vi "Generate Topic Rule Action JSON.vi"(11 "Topic Rule":T1) -> (3 "Action JSON":string)   [LabVIEW 2015, in "NI_AWS_IoT.lvlib"]
uses:
  NI_AWS_IoT.lvlib
  Topic Rule.ctl
  CloudWatch Alarm.ctl
  CloudWatch Metric.ctl
  DynamoDB.ctl
  DynamoDBv2.ctl
  Elasticsearch.ctl
  Firehose.ctl
  Kinesis.ctl
  Lambda.ctl
  Republish.ctl
  S3.ctl
  SNS.ctl
  SQS.ctl
  JSON Parsing/NI_JSON Parsing.lvlib
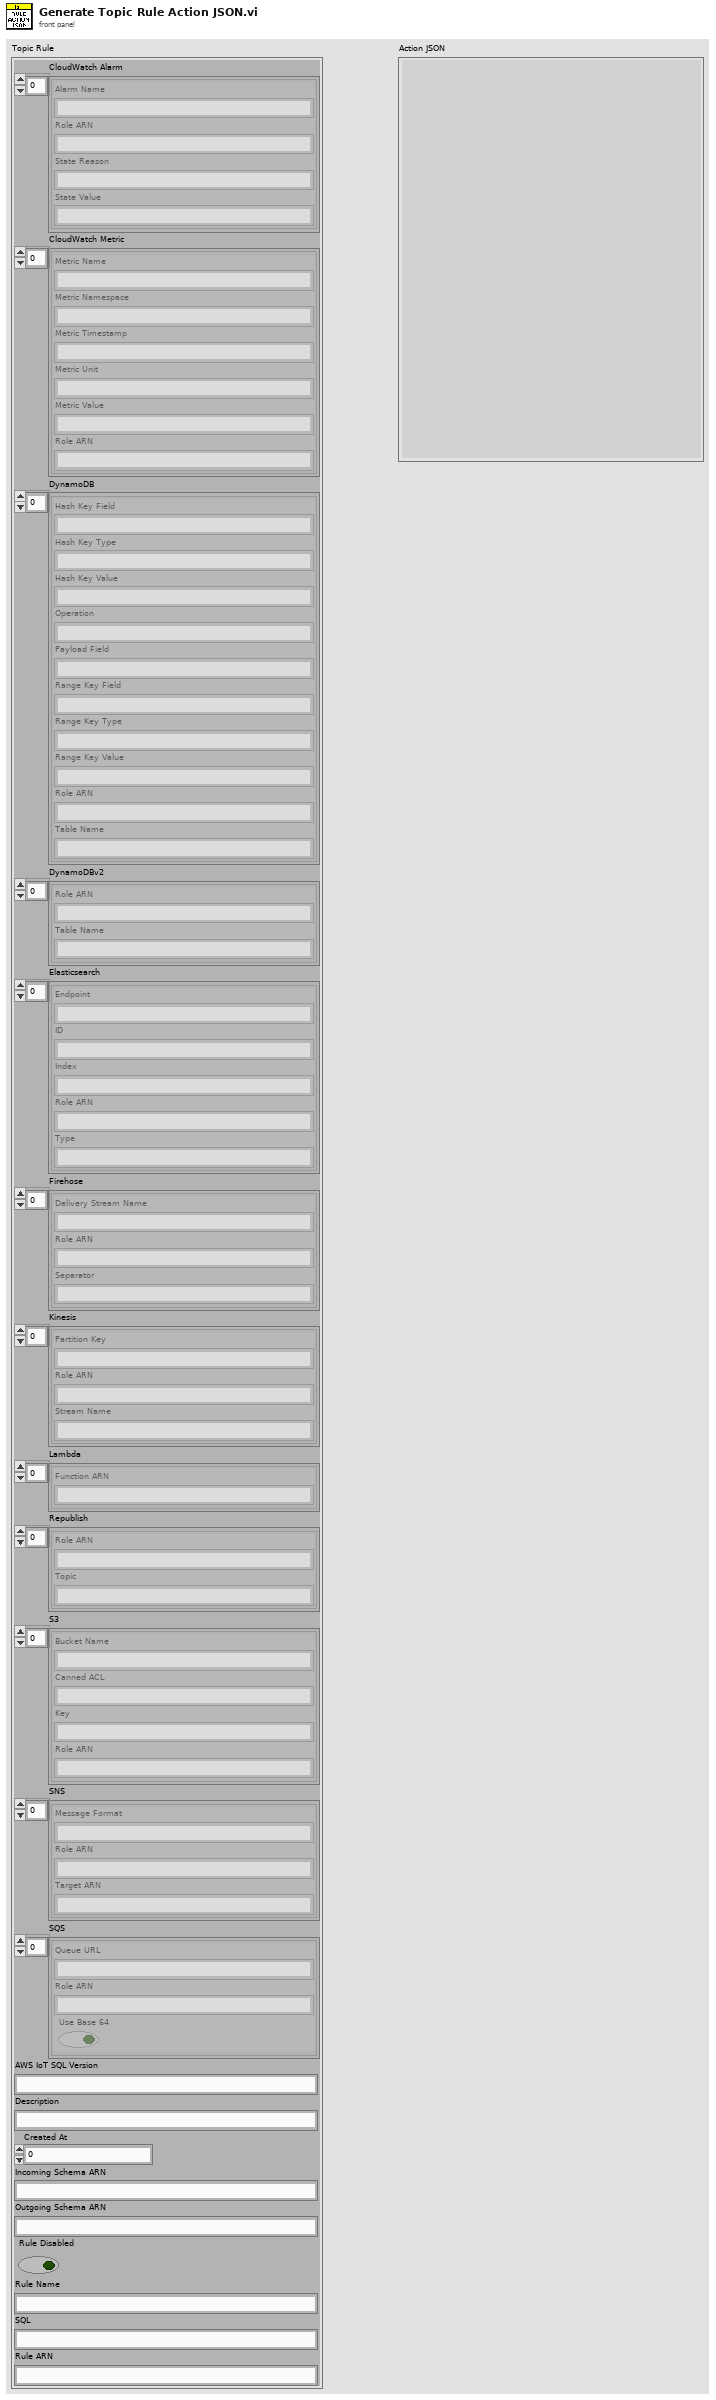
[diagram p1: front panel]
types:
  T1 = typedef "NI_AWS_IoT.lvlib/Topic Rule.ctl" = cluster{"CloudWatch Alarm":T2[], "CloudWatch Metric":T3[], "DynamoDB":T4[], "DynamoDBv2":T5[], "Elasticsearch":T6[], "Firehose":T7[], "Kinesis":T8[], "Lambda":T9[], "Republish":T10[], "S3":T11[], "SNS":T12[], "SQS":T13[], "AWS IoT SQL Version":string, "Description":string, "Created At":u64, "Incoming Schema ARN":string, "Outgoing Schema ARN":string, "Rule Disabled":bool, "Rule Name":string, "SQL":string, "Rule ARN":string}
  T2 = typedef "NI_AWS_IoT.lvlib/CloudWatch Alarm.ctl" = cluster{"Alarm Name":string, "Role ARN":string, "State Reason":string, "State Value":string}
  T3 = typedef "NI_AWS_IoT.lvlib/CloudWatch Metric.ctl" = cluster{"Metric Name":string, "Metric Namespace":string, "Metric Timestamp":string, "Metric Unit":string, "Metric Value":string, "Role ARN":string}
  T4 = typedef "NI_AWS_IoT.lvlib/DynamoDB.ctl" = cluster{"Hash Key Field":string, "Hash Key Type":string, "Hash Key Value":string, "Operation":string, "Payload Field":string, "Range Key Field":string, "Range Key Type":string, "Range Key Value":string, "Role ARN":string, "Table Name":string}
  T5 = typedef "NI_AWS_IoT.lvlib/DynamoDBv2.ctl" = cluster{"Role ARN":string, "Table Name":string}
  T6 = typedef "NI_AWS_IoT.lvlib/Elasticsearch.ctl" = cluster{"Endpoint":string, "ID":string, "Index":string, "Role ARN":string, "Type":string}
  T7 = typedef "NI_AWS_IoT.lvlib/Firehose.ctl" = cluster{"Delivery Stream Name":string, "Role ARN":string, "Separator":string}
  T8 = typedef "NI_AWS_IoT.lvlib/Kinesis.ctl" = cluster{"Partition Key":string, "Role ARN":string, "Stream Name":string}
  T9 = typedef "NI_AWS_IoT.lvlib/Lambda.ctl" = cluster{"Function ARN":string}
  T10 = typedef "NI_AWS_IoT.lvlib/Republish.ctl" = cluster{"Role ARN":string, "Topic":string}
  T11 = typedef "NI_AWS_IoT.lvlib/S3.ctl" = cluster{"Bucket Name":string, "Canned ACL":string, "Key":string, "Role ARN":string}
  T12 = typedef "NI_AWS_IoT.lvlib/SNS.ctl" = cluster{"Message Format":string, "Role ARN":string, "Target ARN":string}
  T13 = typedef "NI_AWS_IoT.lvlib/SQS.ctl" = cluster{"Queue URL":string, "Role ARN":string, "Use Base 64":bool}
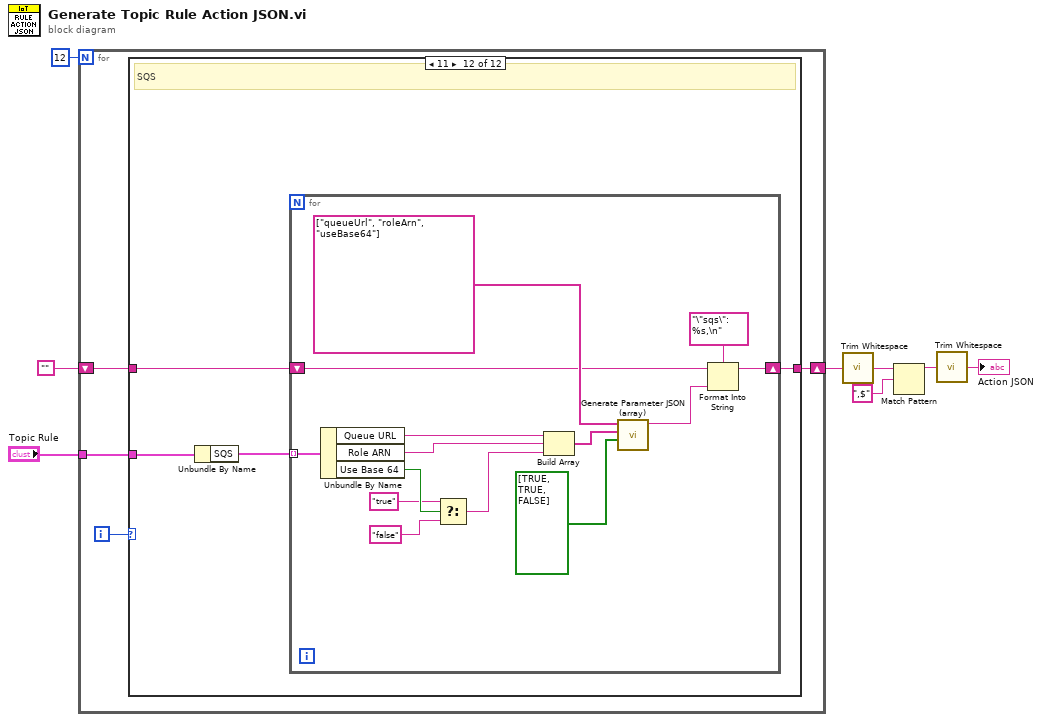
[diagram p0: block diagram]
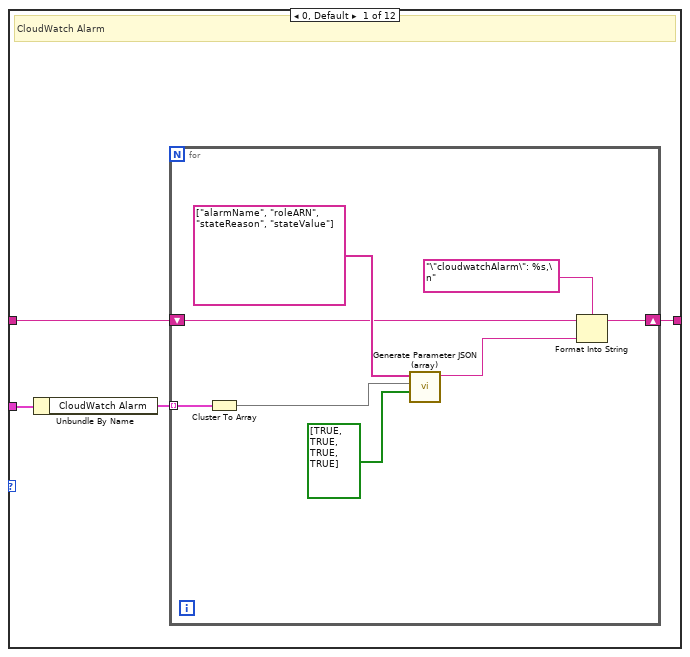
[diagram p2: hidden frame]
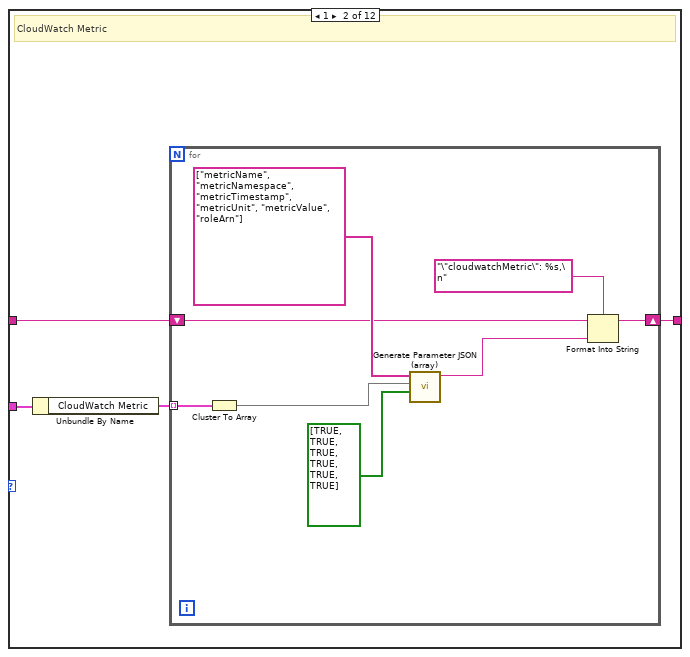
[diagram p3: hidden frame]
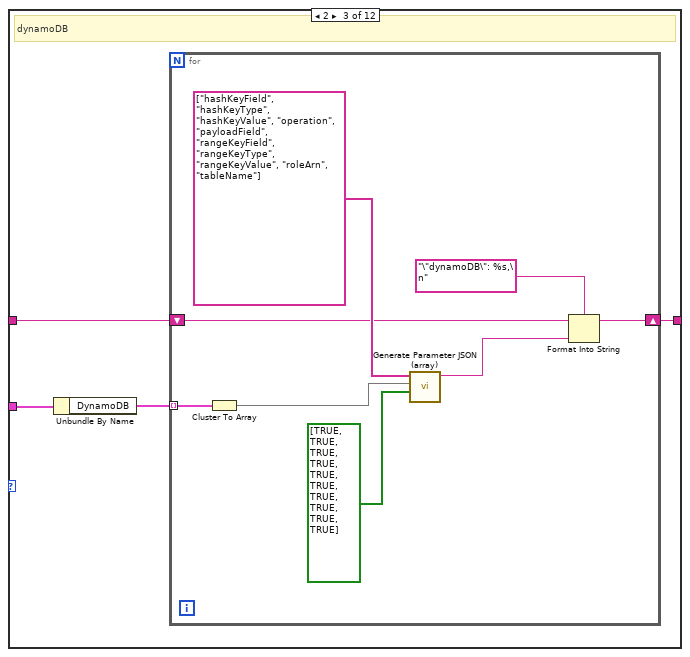
[diagram p4: hidden frame]
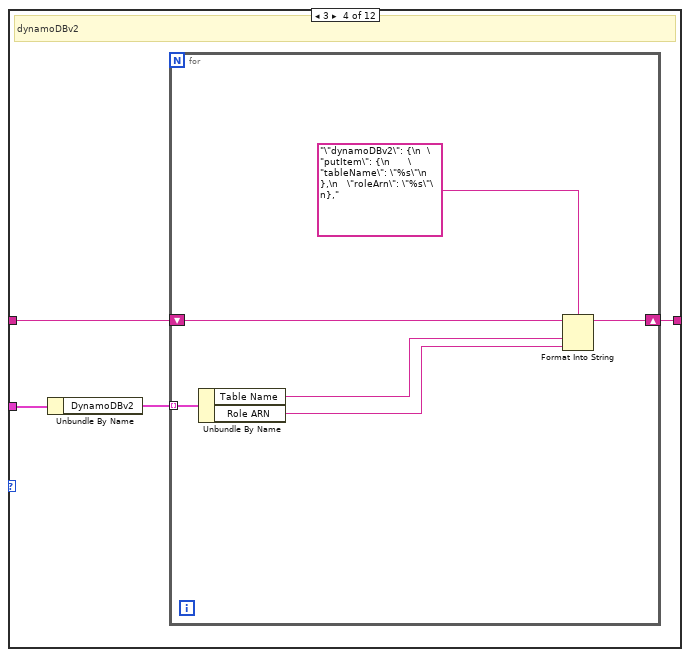
[diagram p5: hidden frame]
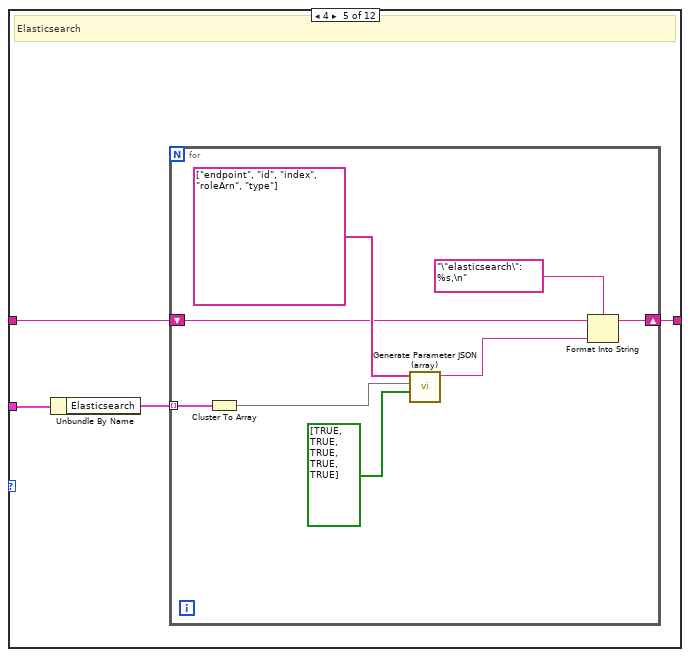
[diagram p6: hidden frame]
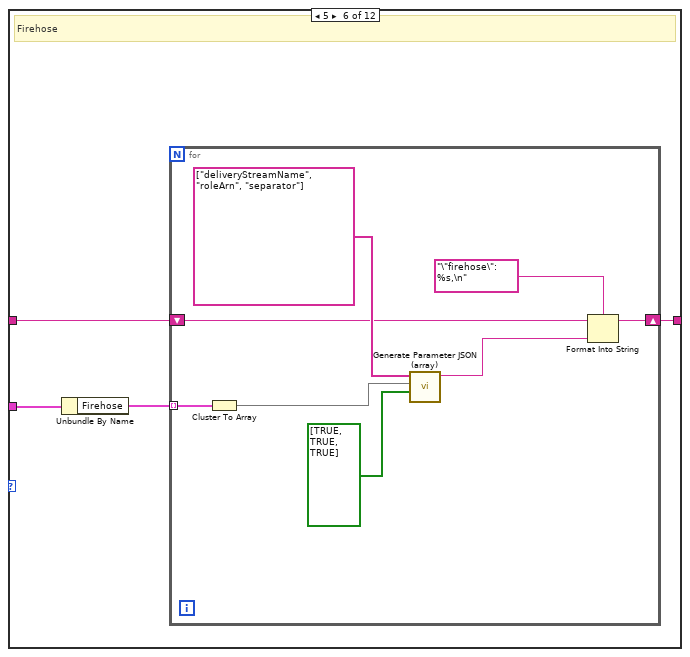
[diagram p7: hidden frame]
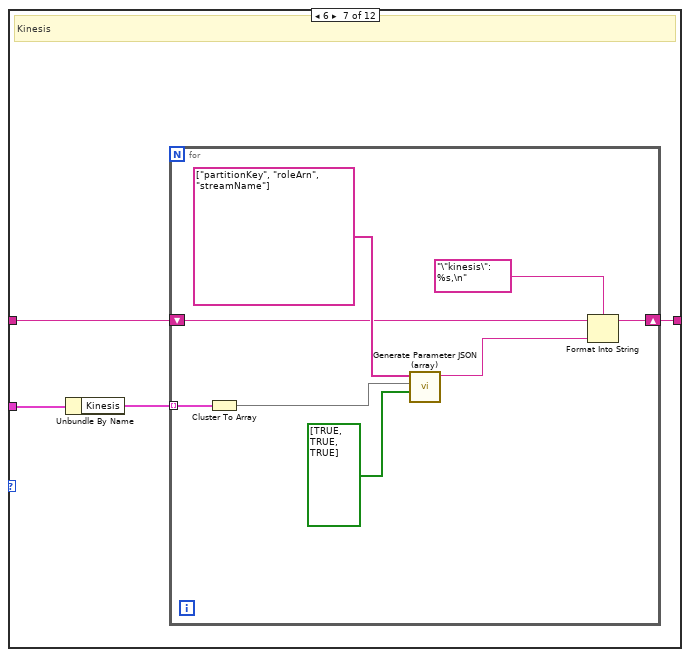
[diagram p8: hidden frame]
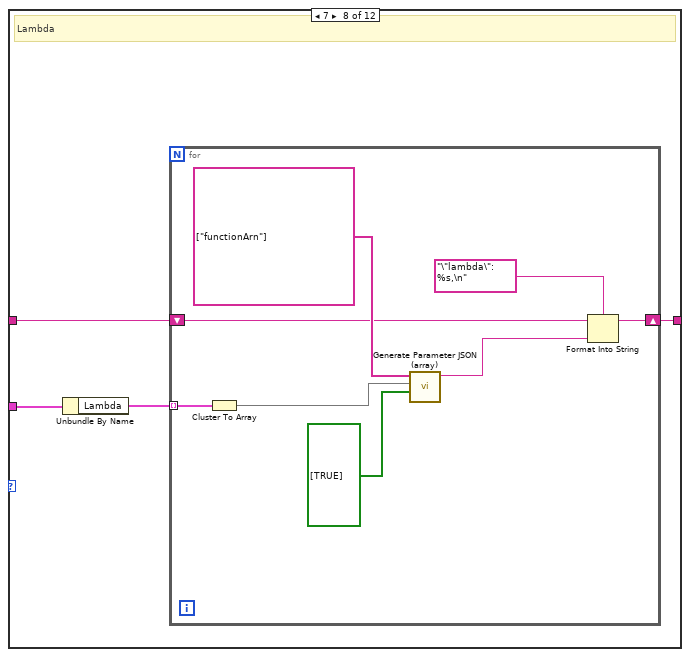
[diagram p9: hidden frame]
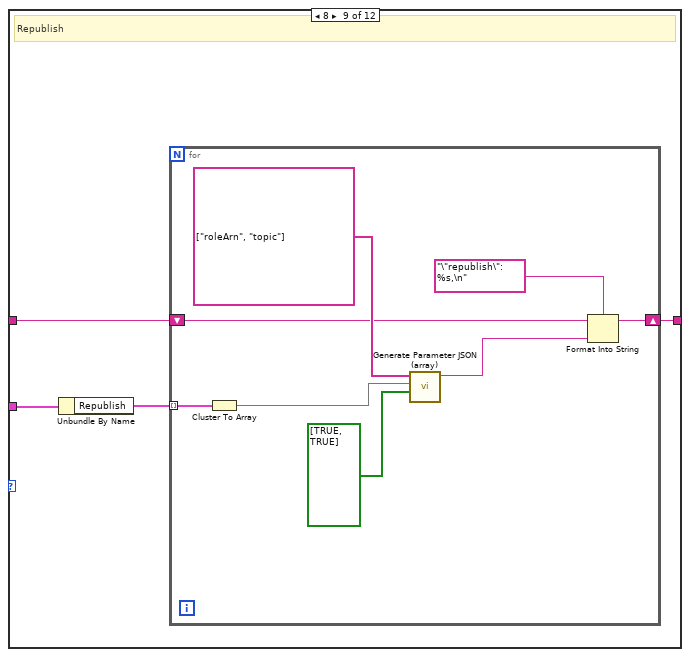
[diagram p10: hidden frame]
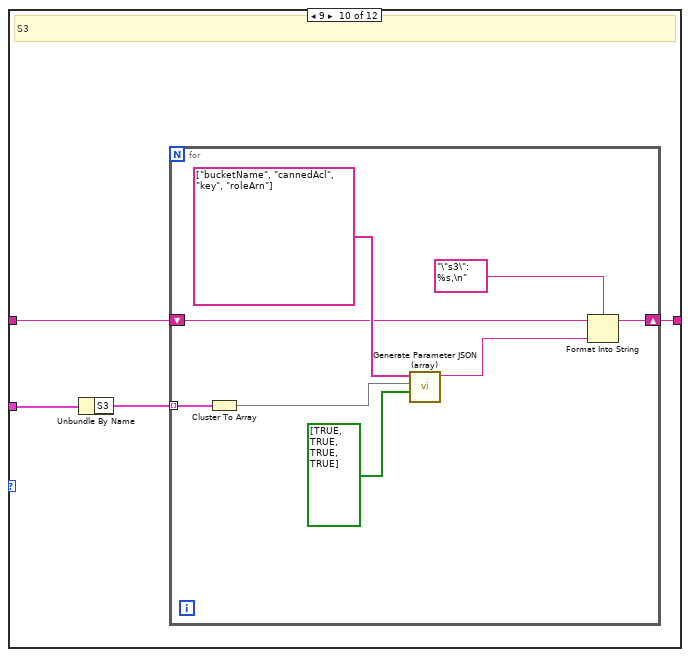
[diagram p11: hidden frame]
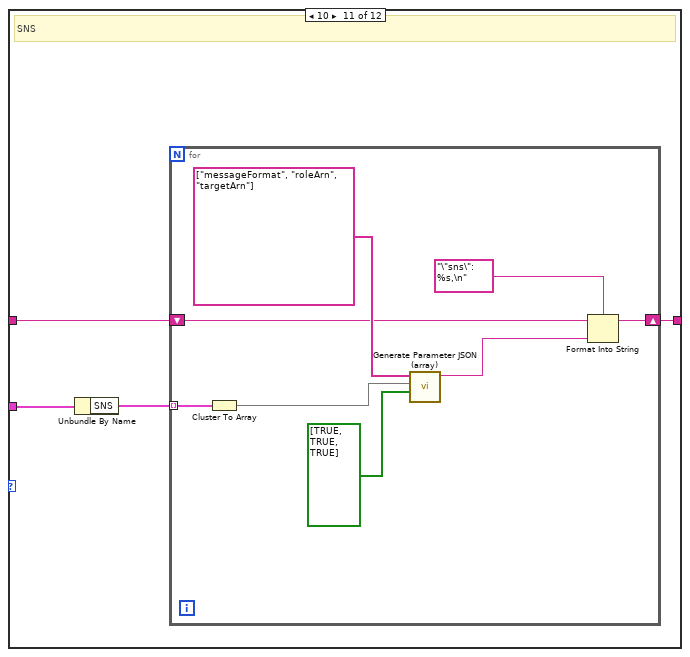
[diagram p12: hidden frame]
diagram:
  n1 = for {
    N: 12 -> [_]
    shift-right: [w9] -> w6
    shift-left: "" -> [w11]
    tunnel: "Topic Rule" -> [w10]
    i -> [w12]
    n2 = case shown="11" w12 {
      tunnel: w11 -> [w14 w26 w38 w50 w60 w72 w84 w96 w108 w120 w132 w144]
      tunnel: w10 -> [w16 w28 w40 w52 w62 w74 w86 w98 w110 w122 w134 w146]
      tunnel: [w13 w25 w37 w49 w59 w71 w83 w95 w107 w119 w131 w143] -> w9
      frame 0, Default {
        # "CloudWatch Alarm"
        n3 = Unbundle By Name(w16) -> ("CloudWatch Alarm"=w15:T2[])
        n4 = for {
          tunnel: w15 -> [w24] mode=indexing
          shift-right: [w19] -> w13
          shift-left: w14 -> [w20]
          n5 = Cluster To Array(cluster=w24) -> (array=w22:string[])
          n6 = call "Generate Parameter JSON (array).vi"("Value in Quotes"=bool[] [TRUE, TRUE, TRUE, TRUE], "Parameter Values"=w22, "Parameter Names"=string[] ["alarmName", "roleARN", "stateReason", "stateValue"]) -> ("Parameter Array JSON"=w17:string)  [unwired: 8 in]
          n7 = Format Into String(format string="\"cloudwatchAlarm\": %s,\n", initial string=w20, w17) -> (resulting string=w19:string)  [unwired: 1 in, 1 out]
        }
      }
      frame 1 {
        # "CloudWatch Metric"
        n8 = Unbundle By Name(w28) -> ("CloudWatch Metric"=w27:T3[])
        n9 = for {
          tunnel: w27 -> [w36] mode=indexing
          shift-right: [w30] -> w25
          shift-left: w26 -> [w32]
          n10 = Cluster To Array(cluster=w36) -> (array=w34:string[])
          n11 = call "Generate Parameter JSON (array).vi"("Value in Quotes"=bool[] [TRUE, TRUE, TRUE, TRUE, TRUE, TRUE], "Parameter Values"=w34, "Parameter Names"=string[] ["metricName", "metricNamespace", "metricTimestamp", "metricUnit", "metricValue", "roleArn"]) -> ("Parameter Array JSON"=w29:string)  [unwired: 8 in]
          n12 = Format Into String(format string="\"cloudwatchMetric\": %s,\n", initial string=w32, w29) -> (resulting string=w30:string)  [unwired: 1 in, 1 out]
        }
      }
      frame 2 {
        # "dynamoDB"
        n13 = Unbundle By Name(w40) -> ("DynamoDB"=w39:T4[])
        n14 = for {
          tunnel: w39 -> [w48] mode=indexing
          shift-right: [w42] -> w37
          shift-left: w38 -> [w44]
          n15 = Cluster To Array(cluster=w48) -> (array=w46:string[])
          n16 = call "Generate Parameter JSON (array).vi"("Value in Quotes"=bool[] [TRUE, TRUE, TRUE, TRUE, TRUE, TRUE, TRUE, TRUE, TRUE, TRUE], "Parameter Values"=w46, "Parameter Names"=string[] ["hashKeyField", "hashKeyType", "hashKeyValue", "operation", "payloadField", "rangeKeyField", "rangeKeyType", "rangeKeyValue", "roleArn", "tableName"]) -> ("Parameter Array JSON"=w41:string)  [unwired: 8 in]
          n17 = Format Into String(format string="\"dynamoDB\": %s,\n", initial string=w44, w41) -> (resulting string=w42:string)  [unwired: 1 in, 1 out]
        }
      }
      frame 3 {
        # "dynamoDBv2"
        n18 = Unbundle By Name(w52) -> ("DynamoDBv2"=w51:T5[])
        n19 = for {
          tunnel: w51 -> [w55] mode=indexing
          shift-right: [w57] -> w49
          shift-left: w50 -> [w58]
          n20 = Unbundle By Name(w55) -> ("Table Name"=w54:string, "Role ARN"=w53:string)
          n21 = Format Into String(format string="\"dynamoDBv2\": {\n  \"putItem\": {\n      \"tableName\": \"%s\"\n   },\n   \"roleArn\": \"%s\"\n},", initial string=w58, w54, w53) -> (resulting string=w57:string)  [unwired: 1 in, 1 out]
        }
      }
      frame 4 {
        # "Elasticsearch"
        n22 = Unbundle By Name(w62) -> ("Elasticsearch"=w61:T6[])
        n23 = for {
          tunnel: w61 -> [w70] mode=indexing
          shift-right: [w64] -> w59
          shift-left: w60 -> [w66]
          n24 = Cluster To Array(cluster=w70) -> (array=w68:string[])
          n25 = call "Generate Parameter JSON (array).vi"("Value in Quotes"=bool[] [TRUE, TRUE, TRUE, TRUE, TRUE], "Parameter Values"=w68, "Parameter Names"=string[] ["endpoint", "id", "index", "roleArn", "type"]) -> ("Parameter Array JSON"=w63:string)  [unwired: 8 in]
          n26 = Format Into String(format string="\"elasticsearch\": %s,\n", initial string=w66, w63) -> (resulting string=w64:string)  [unwired: 1 in, 1 out]
        }
      }
      frame 5 {
        # "Firehose"
        n27 = Unbundle By Name(w74) -> ("Firehose"=w73:T7[])
        n28 = for {
          tunnel: w73 -> [w82] mode=indexing
          shift-right: [w76] -> w71
          shift-left: w72 -> [w78]
          n29 = Cluster To Array(cluster=w82) -> (array=w80:string[])
          n30 = call "Generate Parameter JSON (array).vi"("Value in Quotes"=bool[] [TRUE, TRUE, TRUE], "Parameter Values"=w80, "Parameter Names"=string[] ["deliveryStreamName", "roleArn", "separator"]) -> ("Parameter Array JSON"=w75:string)  [unwired: 8 in]
          n31 = Format Into String(format string="\"firehose\": %s,\n", initial string=w78, w75) -> (resulting string=w76:string)  [unwired: 1 in, 1 out]
        }
      }
      frame 6 {
        # "Kinesis"
        n32 = Unbundle By Name(w86) -> ("Kinesis"=w85:T8[])
        n33 = for {
          tunnel: w85 -> [w94] mode=indexing
          shift-right: [w88] -> w83
          shift-left: w84 -> [w90]
          n34 = Cluster To Array(cluster=w94) -> (array=w92:string[])
          n35 = call "Generate Parameter JSON (array).vi"("Value in Quotes"=bool[] [TRUE, TRUE, TRUE], "Parameter Values"=w92, "Parameter Names"=string[] ["partitionKey", "roleArn", "streamName"]) -> ("Parameter Array JSON"=w87:string)  [unwired: 8 in]
          n36 = Format Into String(format string="\"kinesis\": %s,\n", initial string=w90, w87) -> (resulting string=w88:string)  [unwired: 1 in, 1 out]
        }
      }
      frame 7 {
        # "Lambda"
        n37 = Unbundle By Name(w98) -> ("Lambda"=w97:T9[])
        n38 = for {
          tunnel: w97 -> [w106] mode=indexing
          shift-right: [w100] -> w95
          shift-left: w96 -> [w102]
          n39 = Cluster To Array(cluster=w106) -> (array=w104:string[])
          n40 = call "Generate Parameter JSON (array).vi"("Value in Quotes"=bool[] [TRUE], "Parameter Values"=w104, "Parameter Names"=string[] ["functionArn"]) -> ("Parameter Array JSON"=w99:string)  [unwired: 8 in]
          n41 = Format Into String(format string="\"lambda\": %s,\n", initial string=w102, w99) -> (resulting string=w100:string)  [unwired: 1 in, 1 out]
        }
      }
      frame 8 {
        # "Republish"
        n42 = Unbundle By Name(w110) -> ("Republish"=w109:T10[])
        n43 = for {
          tunnel: w109 -> [w118] mode=indexing
          shift-right: [w112] -> w107
          shift-left: w108 -> [w114]
          n44 = Cluster To Array(cluster=w118) -> (array=w116:string[])
          n45 = call "Generate Parameter JSON (array).vi"("Value in Quotes"=bool[] [TRUE, TRUE], "Parameter Values"=w116, "Parameter Names"=string[] ["roleArn", "topic"]) -> ("Parameter Array JSON"=w111:string)  [unwired: 8 in]
          n46 = Format Into String(format string="\"republish\": %s,\n", initial string=w114, w111) -> (resulting string=w112:string)  [unwired: 1 in, 1 out]
        }
      }
      frame 9 {
        # "S3"
        n47 = Unbundle By Name(w122) -> ("S3"=w121:T11[])
        n48 = for {
          tunnel: w121 -> [w130] mode=indexing
          shift-right: [w124] -> w119
          shift-left: w120 -> [w126]
          n49 = Cluster To Array(cluster=w130) -> (array=w128:string[])
          n50 = call "Generate Parameter JSON (array).vi"("Value in Quotes"=bool[] [TRUE, TRUE, TRUE, TRUE], "Parameter Values"=w128, "Parameter Names"=string[] ["bucketName", "cannedAcl", "key", "roleArn"]) -> ("Parameter Array JSON"=w123:string)  [unwired: 8 in]
          n51 = Format Into String(format string="\"s3\": %s,\n", initial string=w126, w123) -> (resulting string=w124:string)  [unwired: 1 in, 1 out]
        }
      }
      frame 10 {
        # "SNS"
        n52 = Unbundle By Name(w134) -> ("SNS"=w133:T12[])
        n53 = for {
          tunnel: w133 -> [w142] mode=indexing
          shift-right: [w136] -> w131
          shift-left: w132 -> [w138]
          n54 = Cluster To Array(cluster=w142) -> (array=w140:string[])
          n55 = call "Generate Parameter JSON (array).vi"("Value in Quotes"=bool[] [TRUE, TRUE, TRUE], "Parameter Values"=w140, "Parameter Names"=string[] ["messageFormat", "roleArn", "targetArn"]) -> ("Parameter Array JSON"=w135:string)  [unwired: 8 in]
          n56 = Format Into String(format string="\"sns\": %s,\n", initial string=w138, w135) -> (resulting string=w136:string)  [unwired: 1 in, 1 out]
        }
      }
      frame 11 {
        # "SQS"
        n57 = Unbundle By Name(w146) -> ("SQS"=w145:T13[])
        n58 = for {
          tunnel: w145 -> [w154] mode=indexing
          shift-right: [w156] -> w143
          shift-left: w144 -> [w158]
          n59 = Unbundle By Name(w154) -> ("Queue URL"=w153:string, "Role ARN"=w151:string, "Use Base 64"=w150:bool)
          n60 = Select(t="true", s=w150, f="false") -> (s? t:f=w147:string)
          n61 = Build Array(w153, w151, w147) -> (w152:string[])
          n62 = call "Generate Parameter JSON (array).vi"("Value in Quotes"=bool[] [TRUE, TRUE, FALSE], "Parameter Values"=w152, "Parameter Names"=string[] ["queueUrl", "roleArn", "useBase64"]) -> ("Parameter Array JSON"=w155:string)  [unwired: 8 in]
          n63 = Format Into String(format string="\"sqs\": %s,\n", initial string=w158, w155) -> (resulting string=w156:string)  [unwired: 1 in, 1 out]
        }
      }
    }
  }
  n64 = call <vilib>:"Trim Whitespace.vi"("string"=w6) -> ("trimmed string"=w4:string)  [unwired: 1 in]
  n65 = Match Pattern(string=w4, regular expression=",$") -> (before substring=w2:string)  [unwired: 1 in, 3 out]
  n66 = call <vilib>:"Trim Whitespace.vi"("string"=w2) -> ("trimmed string"=→"Action JSON":string)  [unwired: 1 in]
